vi "Read Matlab Params.vi"(8 "error in (no error)":errorcluster, 10 "Enum":T1(ring), 11 "TrialBasedExperiment in":refnum<class "WhiteNoiseOrientationDetection.lvclass">) -> (0 "error out":errorcluster, 2 "Matlab Param Array":cluster{"Name":string, "Data":variant}[](array[cluster]), 3 "TrialBasedExperiment out":refnum<class "WhiteNoiseOrientationDetection.lvclass">)   [LabVIEW 2014, in "WhiteNoiseOrientationDetection.lvclass"]
uses:
  WhiteNoiseOrientationDetection.lvclass
  WhiteNoiseOrientationDetection.lvclass/WhiteNoiseOrientationDetection.ctl
  Trial Based Experiment Statechart/MatlabExperiment/MatlabExperiment.lvclass
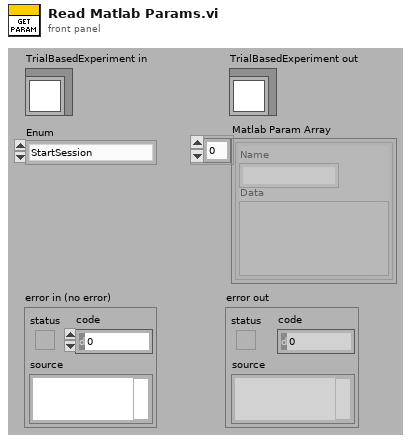
[diagram p1: front panel]
types:
  T1 = enum16{"StartSession", "StartTrial", "ShowStimulus"}
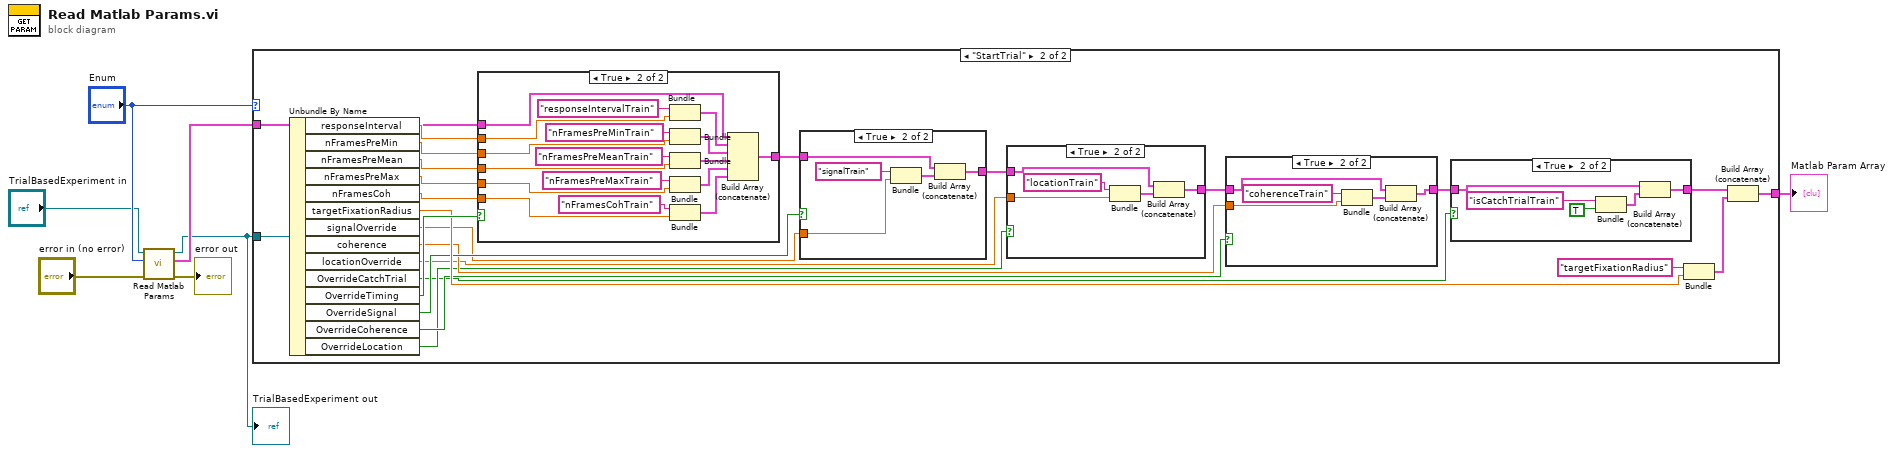
[diagram p0: block diagram]
diagram:
  n1 = call-parent "Read Matlab Params.vi"("error in (no error)"="error in (no error)", "Enum"="Enum", "TrialBasedExperiment in"="TrialBasedExperiment in") -> ("error out"=→"error out":errorcluster, "Matlab Param Array"=w5:cluster{"Name":string, "Data":variant}[], "TrialBasedExperiment out"=w1:refnum<class "WhiteNoiseOrientationDetection.lvclass">)  [unwired: 6 in]
  "TrialBasedExperiment out" <- w1
  n2 = case shown="\"StartTrial\"" "Enum" {
    tunnel: w1 -> [_ w32]
    tunnel: w5 -> [w8 w30]
    tunnel: [w8 w22] -> w2
    frame "StartSession", Default {
    }
    frame "StartTrial" {
      n3 = Unbundle By Name(w32) -> ("responseInterval"=w31:dbl, "nFramesPreMin"=w29:dbl, "nFramesPreMean"=w28:dbl, "nFramesPreMax"=w27:dbl, "nFramesCoh"=w26:dbl, "targetFixationRadius"=w23:dbl, "signalOverride"=w15:dbl, "coherence"=w16:dbl, "locationOverride"=w9:dbl, "OverrideCatchTrial"=w10:bool, "OverrideTiming"=w25:bool, "OverrideSignal"=w21:bool, "OverrideCoherence"=w17:bool, "OverrideLocation"=w13:bool)
      n4 = case shown="True" w25 {
        tunnel: w31 -> [_ w73]
        tunnel: w30 -> [w57 w71]
        tunnel: [w57 w70] -> w20
        tunnel: w29 -> [_ w65]
        tunnel: w28 -> [_ w64]
        tunnel: w27 -> [_ w63]
        tunnel: w26 -> [_ w62]
        frame False {
        }
        frame True {
          n5 = Bundle("responseIntervalTrain", "responseInterval"=w73) -> (w72:cluster{string, "responseInterval":dbl})  [unwired: 1 out]
          n6 = Bundle("nFramesPreMinTrain", "nFramesPreMin"=w65) -> (w61:cluster{string, "nFramesPreMin":dbl})  [unwired: 1 out]
          n7 = Bundle("nFramesPreMeanTrain", "nFramesPreMean"=w64) -> (w60:cluster{string, "nFramesPreMean":dbl})  [unwired: 1 out]
          n8 = Bundle("nFramesPreMaxTrain", "nFramesPreMax"=w63) -> (w59:cluster{string, "nFramesPreMax":dbl})  [unwired: 1 out]
          n9 = Bundle("nFramesCohTrain", "nFramesCoh"=w62) -> (w58:cluster{string, "nFramesCoh":dbl})  [unwired: 1 out]
          n10 = Build Array (concatenate)(w71, w72, w61, w60, w59, w58) -> (w70:cluster{"Name":string, "Data":variant}[])
        }
      }
      n11 = case shown="True" w21 {
        tunnel: [w51 w56] -> w12
        tunnel: w20 -> [w51 w54]
        tunnel: w15 -> [_ w53]
        frame False {
        }
        frame True {
          n12 = Bundle("signalTrain", "signalOverride"=w53) -> (w52:cluster{string, "signalOverride":dbl})  [unwired: 1 out]
          n13 = Build Array (concatenate)(w54, w52) -> (w56:cluster{"Name":string, "Data":variant}[])
        }
      }
      n14 = case shown="True" w13 {
        tunnel: [w33 w38] -> w11
        tunnel: w12 -> [w33 w35]
        tunnel: w9 -> [_ w34]
        frame False {
        }
        frame True {
          n15 = Bundle("locationTrain", "locationOverride"=w34) -> (w36:cluster{string, "locationOverride":dbl})  [unwired: 1 out]
          n16 = Build Array (concatenate)(w35, w36) -> (w38:cluster{"Name":string, "Data":variant}[])
        }
      }
      n17 = case shown="True" w17 {
        tunnel: [w45 w50] -> w19
        tunnel: w11 -> [w45 w48]
        tunnel: w16 -> [_ w47]
        frame False {
        }
        frame True {
          n18 = Bundle("coherenceTrain", "coherence"=w47) -> (w46:cluster{string, "coherence":dbl})  [unwired: 1 out]
          n19 = Build Array (concatenate)(w48, w46) -> (w50:cluster{"Name":string, "Data":variant}[])
        }
      }
      n20 = case shown="True" w10 {
        tunnel: [w39 w44] -> w18
        tunnel: w19 -> [w39 w42]
        frame False {
        }
        frame True {
          n21 = Bundle("isCatchTrialTrain", TRUE) -> (w41:cluster{string, bool})  [unwired: 1 out]
          n22 = Build Array (concatenate)(w42, w41) -> (w44:cluster{"Name":string, "Data":variant}[])
        }
      }
      n23 = Bundle("targetFixationRadius", "targetFixationRadius"=w23) -> (w14:cluster{string, "targetFixationRadius":dbl})  [unwired: 1 out]
      n24 = Build Array (concatenate)(w18, w14) -> (w22:cluster{"Name":string, "Data":variant}[])
    }
  }
  "Matlab Param Array" <- w2
